vi "Odbiór UDP z SbRIO.vi"(5 "Queue B in":T1, 8 "error in udp (no error)":errorcluster, 11 "port":refnum<k16>) -> (0 "error out udp":errorcluster, 1 "error out variant":errorcluster, 3 "UDP Network Connection out":refnum<k16>)   [LabVIEW 2015]
uses:
  QMH Fundamentals - Message Cluster.ctl
  RT/CANFrameControl.ctl
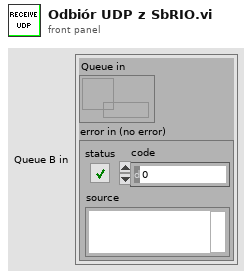
[diagram p1: front panel]
types:
  T1 = cluster{"Queue in":refnum<queue>, "error in (no error)":errorcluster}
  T2 = typedef "CANFrameControl.ctl" = cluster{"identifier":u32, "extended?":bool, "type":u8, "payload":u8[]}
  T3 = cluster{"CAN frame":T2, "GPS Data":cluster{"Oldest Read Timestamp":timestamp, "Latitude":dbl, "Longitude":dbl, "Speed over Ground (Knots)":dbl, "True Track Angle (Deg)":dbl, "Altitude Above Mean Sea Level":dbl, "number of satellites in view.number of satellites":i8, "Fix Quality ":u16}}
  T4 = typedef "QMH Fundamentals - Message Cluster.ctl" = cluster{"Message":string, "Message Data":variant}
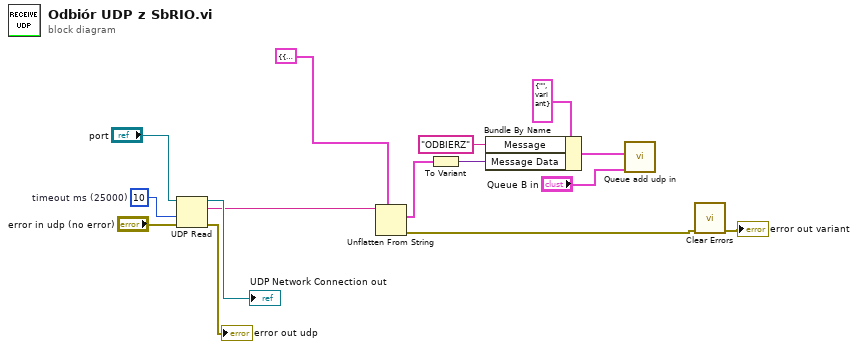
[diagram p0: block diagram]
diagram:
  w15 = 10  # timeout ms (25000)
  n1 = UDP Read(connection ID="port", timeout ms (25000)=w15, 8:"error in udp (no error)") -> (data out=w7:string, error out=→"error out udp":errorcluster, 3:→"UDP Network Connection out":refnum<k16>)  [unwired: 1 in, 2 out]
  n2 = Unflatten From String(type=T3 {"CAN frame"={"identifier"=0, "extended?"=FALSE, "type"=0, "payload"=[]}, "GPS Data"={"Oldest Read Timestamp"=timestamp(0 s since 1904-01-01), "Latitude"=0.0, "Longitude"=0.0, "Speed over Ground (Knots)"=0.0, "True Track Angle (Deg)"=0.0, "Altitude Above Mean Sea Level"=0.0, "number of satellites in view.number of satellites"=0, "Fix Quality "=0}} ("output cluster"), binary string=w7) -> (value=w12:T3, error out=w5:errorcluster)  [unwired: 3 in, 1 out]
  n3 = To Variant(anything=w12) -> (Variant=w11:variant)
  n4 = Bundle By Name(cluster=T4 {"Message"="", "Message Data"=variant} ("Message Cluster"), "Message"="ODBIERZ", "Message Data"=w11) -> (w3:T4)
  n5 = call "Queue add udp in.vi"("Queue B in"="Queue B in", "Message Cluster"=w3) -> ()  [unwired: 10 in]
  n6 = call <vilib>:"Clear Errors.vi"("error in (no error)"=w5) -> ("error out"=→"error out variant":errorcluster)  [unwired: 5 in, 1 out]
